vi "Robot Global Data.vi"() -> ()   [LabVIEW 2015]
doc: "This global VI can contain as many global variables as you need. Place a control on the panel, give it a good name. To read or write to it from a VI, drag the icon to the diagram of that VI. You can also drag from the project. Click on the node to change which global you access. You shouldn't have multiple locations writing to a global or it will cause a race-condition."
uses:
  <vilib>/Rock Robotics/WPI/Camera/WPI_CameraImageSize.ctl
  <vilib>/Rock Robotics/WPI/DriverStation/WPI_DriverStationRobotMode2.ctl
  Common Code/Auton Command Cluster.ctl
  Common Code/Drivetrain Status Cluster.ctl
  Common Code/Drivetrain Modes.ctl
  Common Code/Dist Drive Status.ctl
  Common Code/Dashboard Communication/Dashboard Display Data.ctl
  Common Code/Auton File Lists.ctl
  Common Code/Encoder Values Super Cluster.ctl
  Common Code/Encoder Values.ctl
  Common Code/IMU Data.ctl
  navX-MXP Library/COMMON/TypeDefs/Value TypeDefs/navX NAVX_CAL_STATUS.ctl
  navX-MXP Library/COMMON/TypeDefs/Value TypeDefs/navX NAVX_OP_STATUS.ctl
  Common Code/Power and Diagnostic Data.ctl
  Common Code/Utilities/PDP Data.ctl
  Common Code/Utilities/PCM Data.ctl
  Common Code/Shooter State Cluster.ctl
  Common Code/Shooter State.ctl
  Common Code/Shoot Modes Enum.ctl
  Common Code/Shot Type.ctl
  Common Code/Intake Status Cluster.ctl
  Common Code/Intake Mode.ctl
  Common Code/Intake States.ctl
  Common Code/Ultrasonic Data.ctl
  Common Code/Climb Status Cluster.ctl
  Common Code/Major Loop Times.ctl
  Common Code/Dashboard Communication/Dashboard Control Data.ctl
  Common Code/Shooter Presets.ctl
  Common Code/Shot Presets.ctl
  Common Code/Encoder Control.ctl
  Common Code/Drivetrain Settings.ctl
  Common Code/Goal Vision Packet.ctl
  Common Code/Dashboard Drivetrain Command.ctl
  Common Code/Drivetrain Vision.ctl
  Common Code/Ball Tracking Command Cluster.ctl
  Common Code/Ball Vision Packet.ctl
  Common Code/Tracking Mode.ctl
  Common Code/Intake Presets.ctl
  Common Code/Drivetrain Output Range.ctl
  Common Code/IntakeEcoderControl.ctl
  Common Code/Climb Presets.ctl
  Common Code/Shooter Command Cluster.ctl
  Common Code/Shooter Commands.ctl
  Common Code/Climb Command Cluster.ctl
  Common Code/Climb Mode.ctl
  Common Code/Climb Manual State.ctl
  Common Code/Drivetrain Commands.ctl
  Common Code/Manual Shoot.ctl
  Common Code/Intake Commands Cluster.ctl
  Common Code/Intake Commands.ctl
  Common Code/Manual Intake Commands.ctl
  Common Code/Keyboard Packet.ctl
  navX-MXP Library/navX-MXP IMU.lvlib
panel:
  in  "Right RPM":dbl
  in  "Left RPM":dbl
  out "Auton File Loop Timer":u32
  out "US Loop Timer":u32
  out "Intake Loop Timer":u32
  out "Shooter Loop Timer":u32
  out "DT Loop Timer":u32
  out "Climb Status Cluster":T1
  out "Ultrasonic Data":T2
  in  "Keyboard Cluster":T3
  out "Shooter State":T4 {"Trigger Output" scale=-1.0..1.0; "Angle Motor Output" scale=-1.0..1.0; "Right RPM" scale=0.0..5000.0; "Left RPM" scale=0.0..5000.0}
  in  "Intake Status Cluster":T8={"Roller Power"=0.0, "Angle Power"=0.0, "Intake Mode"=enum."Auto", "Intake States"=enum."Idle", "Rollers Active?"=FALSE, "Current Height"=0.0, "Target Height"=0.0, "Encoder Raw Position"=0.0, "Forward Tripped?"=FALSE, "Backward Tripped?"=FALSE, "Override IR?"=FALSE}
  out "Is IMU Reset?":bool
  in  "Reset IMU":bool
  in  "Boolean":bool
  in  "Intake Commands Cluster":T11={"Intake Commands"=enum."Load", "Intake Mode"=enum."Auto", "Override IR"=FALSE}
  in  "Manual Intake Commands":T13
  in  "Queue File Names":string[](array[string])
  in  "NavX Opened":bool
  in  "IMU Yaw Zero":dbl
  in  "IMU Roll Zero":dbl
  in  "IMU Pitch Zero":dbl
  in  "Manual Shoot":T14
  out "IMU Data":T15 {"NAVX_OP_STATUS" items=["INITIALIZING", "SELFTEST_IN_PROGRESS", "ERROR", "IMU_AUTOCAL_IN_PROGRESS", "NORMAL"]; "NAVX_CAL_STATUS" items=["IMU_CAL_STATE_MASK"=3, "IMU_CAL_INPROGRESS"=0, "IMU_CAL_ACCUMULATE"=1, "IMU_CAL_COMPLETE"=2, "MAG_CAL_COMPLETE"=4, "BARO_CAL_COMPLETE"=8]}
  in  "Right Pot 0":dbl
  in  "Left Pot 0":dbl
  out "Encoder Values":T18
  in  "Dashboard Drivetrain Command":T20
  out "General Scripts":string
  in  "Auton File Lists":T22
  in  "Current Auton Command Data":T23
  in  "Dashboard Packet":T24={"Shooter Presets"={"Batter Shot"={"Left Wheel RPM"=0.0, "Right Wheel RPM"=0.0, "Angle"=0.0}, "Deep Middle Shot"={"Left Wheel RPM"=0.0, "Right Wheel RPM"=0.0, "Angle"=0.0}, "Manual Shot"={"Left Wheel RPM"=0.0, "Right Wheel RPM"=0.0, "Angle"=0.0}, "Left Ticks Per Rotation"=0.0, "Right Ticks Per Rotation"=0.0, "Low Bar Shot"={"Left Wheel RPM"=0.0, "Right Wheel RPM"=0.0, "Angle"=0.0}, "Shooter RPM Tolerance"=0.0, "IIR Filter Power"=0.0, "Trigger Power"=0.0, "Fire from Load Delay"=0, "Angle Pot M"=0.0, "Angle Pot B"=0.0, "Shooter Length"=0.0, "String Pot Dist"=0.0, "Angle PID gains"={"proportional gain (Kc)"=1.0, "integral time (Ti, min)"=0.01, "derivative time (Td, min)"=0.0}, "Angle Motor Output"={"output high"=0.0, "output low"=0.0}, "Shooter Angle Tolerance"=0.0, "Vision Shoot x^2"=0.0, "Vision Shoot x"=0.0, "Dist from Axis Cam to Pivot"=0.0, "High Goal Center Height"=97.0, "Feed Forward Max Accel"=0.0, "Feed Forward Kv"=0.0, "Backwards Trigger"=0.0, "Shot Finish Delay (ms)"=0.0, "Angle Max Current"=0.0, "Angle Current Trip Time"=0.0, "Shooter Intake Angle"=0.0, "Vision Shoot c"=0.0, "Reset?"=FALSE, "Servo Release Delay"=0.0, "Servo Idle Angle"=0, "Servo Hold Angle"=0, "Angle Pot x^2"=0.0, "Angle Pot x"=0.0, "Angle Pot c"=0.0, "Ignore Angle?"=FALSE}, "Encoder Control"={"Right Tick Constant"=0.0, "Left Tick Constant"=0.0, "Reset?"=FALSE, "Y Dist"={"PID gains"={"proportional gain (Kc)"=0.0, "integral time (Ti, min)"=0.0, "derivative time (Td, min)"=0.0}}, "Y Stop Thresh"=0.0, "Y Stop Speed"=0.0}, "Steer PID output"={"output high"=0.0, "output low"=0.0}, " Steer PID gains"={"proportional gain (Kc)"=0.0, "integral time (Ti, min)"=0.0, "derivative time (Td, min)"=0.0}, "Drivetrain Settings"={"Gyro Tolerance"=0.0, "Throttle Ramp (ms)"=0.0, "Angular rate compensation"=FALSE, "Throttle to Rate Scale"=1.0, "Rate compensation gain"=0.01, "Kv"=0.0, "Ka"=0.0, "Feed Forward P"=0.0, "Feed Forward D"=0.0, "Goal Vision PID gains"={"proportional gain (Kc)"=1.0, "integral time (Ti, min)"=0.01, "derivative time (Td, min)"=0.0}, "Goal Detection Window"=0.0}, "Vision Packet"={"Distance"=0.0, "Center X"=0.0, "Center Y"=0.0, "Found Target?"=FALSE}, "Dashboard Drivetrain Command"={"Drivetrain Vision"={"Goal Window"=0.0, "Ball Window"=0.0}}, "Info/Command Cluster"={"Distance to Ball"=0.0, "Desired Angle"=0.0, "Command"=enum."Turn to Ball", "Pixels from Center"=0.0}, "Ball Vision Packet"={"Ball Detected?"=FALSE, "Distance to Ball"=0.0, "Desired Angle"=0.0, "Pixels from Center"=0.0, "Tracking mode"=enum."Turn to Ball"}, "Intake Presets"={"Intake Speed"=0.0, "Outake Speed"=0.0, "Low Height"=0.0, "Half Height"=0.0, "Full Height"=0.0, "Angle Speed"=0.0, "Fast Angle"=0.0, "Encoder Scale"=0.0, "Load Height"=0.0, "Output Range"={"output high"=0.0, "output low"=0.0}, "Rotation Power Max/Min"=0.0, "MaxCurrent"=0.0, "Intake Trip Time"=0.0, "Idle Height"=0.0, "Max Height"=0.0, "Reset Encoders?"=FALSE, "PID gains"={"proportional gain (Kc)"=0.0, "integral time (Ti, min)"=0.0, "derivative time (Td, min)"=0.0}}, "Intake Encoder Control"={"Arm Tick Constant"=0.0, "Reset?"=FALSE, "Y Dist"={"PID gains"={"proportional gain (Kc)"=0.0, "integral time (Ti, min)"=0.0, "derivative time (Td, min)"=0.0}}, "Y Stop Thresh"=0.0, "Y Stop Speed"=0.0}, "Climb Presets"={"Pull Power"=0.0, "Unpin Power"=0.0, "Time to Hold"=0.0}, "Ultrasonic Limit"=0.0, "Roll Limit"=0.0, "Pitch Limit"=0.0, "Goal Output Range"={"output high"=0.0, "output low"=0.0}} {"Intake Presets"."Max Height" format="%#_7g"; "Intake Presets"."Rotation Power Max/Min" format="%#_7g"; "Drivetrain Settings"."Goal Vision PID gains"."derivative time (Td, min)" format="%.3f"; "Drivetrain Settings"."Goal Vision PID gains"."integral time (Ti, min)" format="%.3f"; "Drivetrain Settings"."Goal Vision PID gains"."proportional gain (Kc)" format="%.3f"}
  out "Driver Station IP":dbl
  in  "Auton File Index":i32
  in  "Auton Field Index":i32
  out "Dashboard Status Data":T37={"Auton Command Cluster"={"Command ID"=0, "maxTime"=0.0, "Y Distance"=0.0, "Heading"=0.0, "Throttle"=0.0, "Async"=0.0, "Velocity"=0.0, "Acceleration"=0.0, "To"=0.0, "Condition"=0.0, "Shot Type"=0.0, "Left RPM"=0.0, "Override RPM"=0, "Override Angle"=0, "Right RPM"=0.0, "Angle"=0.0, "Intake Mode"=0, "Intake Cmd"=0, "Intake O"=0, "Eject O"=0, "Angle O"=0, "Arm O"=0, "Intake Speed"=0.0, "Eject Speed"=0.0, "Arm Angle"=0.0, "Arm Speed"=0.0, "Intake?"=0, "Eject?"=0}, "Auton File Lists"={"Current Queue"="", "General Scripts"="", "Defense Scripts"="", "Movement Scripts"=""}, "Drivetrain Status Cluster"={"Modes"=enum."Climb", "Y (Throttle)"=0.0, "X (Steer)"=0.0, "Gyro In Range?"=FALSE, "Distance Drive Finished?"=FALSE, "Stop Eject Lockout"=FALSE, "Dist Drive Status"={"Y In Range"=FALSE, "X In Range"=FALSE, "Gyro In Range"=FALSE, "Y Dist"=0.0, "X Dist"=0.0, "Gyro"=0.0}, "Y Target"=0.0, "Heading Target"=0.0, "Vision Target Aligned?"=FALSE, "Gear"=0.0, "1st Gear Time"=0.0, "2nd Gear Time"=0.0, "1st Gear Shifts"=0.0, "2nd Gear Shifts"=0.0}, "Encoder Values"={"Left Encoder"={"Distance"=0.0, "Speed"=0.0, "Ticks"=0.0}, "Right Encoder"={"Distance"=0.0, "Speed"=0.0, "Ticks"=0.0}}, "IMU Data"={"Pitch"=0.0, "Roll"=0.0, "Yaw"=0.0, "Data Valid?"=FALSE, "Temp"=0.0, "MOVING"=FALSE, "YAW_STABLE"=FALSE, "Accel X"=0.0, "Accel Y"=0.0, "Accel Z"=0.0, "Accel Magnitude"=0.0, "Pitch Rate"=0.0, "Roll Rate"=0.0, "Yaw Rate"=0.0, "NavX Opened?"=FALSE, "NAVX_CAL_STATUS"=0, "NAVX_OP_STATUS"=0}, "Power and Diagnostic Data"={"PDP Data"={"Battery Voltage"=0.0, "Temperature (degrees C)"=0.0, "Internal Battery R (Ohms)"=0.0, "Energy (J)"=0.0, "Power (W)"=0.0, "Total Current (A)"=0.0, "Battery Voltage Fault"=FALSE, "Temperature Fault"=FALSE, "Hardware Fault"=FALSE, "Currents"={"[0]"=0.0, "[1]"=0.0, "[2]"=0.0, "[3]"=0.0, "[4]"=0.0, "[5]"=0.0, "[6]"=0.0, "[7]"=0.0, "[8]"=0.0, "[9]"=0.0, "[10]"=0.0, "[11]"=0.0, "[12]"=0.0, "[13]"=0.0, "[14]"=0.0, "[15]"=0.0}, "Current Faults"={"[0]"=FALSE, "[1]"=FALSE, "[2]"=FALSE, "[3]"=FALSE, "[4]"=FALSE, "[5]"=FALSE, "[6]"=FALSE, "[7]"=FALSE, "[8]"=FALSE, "[9]"=FALSE, "[10]"=FALSE, "[11]"=FALSE, "[12]"=FALSE, "[13]"=FALSE, "[14]"=FALSE, "[15]"=FALSE}}, "PCM Data"={"Compressor Fault"=FALSE, "Solenoid Fault"=FALSE, "Compressor Enabled"=FALSE, "Hardware Fault"=FALSE, "Compressor Current"=0.0}, "roboRIO input voltage (V)"=0.0, "roboRIO input current (A)"=0.0, "3.3V Rail Short"=FALSE, "5 V Rail Short"=FALSE, "6 V Rail Short"=FALSE, "roboRIO Brownout"=FALSE, "Outputs Enabled?"=FALSE}, "Gyro"=0.0, "Shooter State Cluster"={"State"=enum."Idle", "Left RPM"=0.0, "Right RPM"=0.0, "Shooter Ready?"=FALSE, "Ball Loaded?"=FALSE, "Current Angle"=0.0, "Angle Motor Output"=0.0, "Trigger Output"=0.0, "Angle Ready?"=FALSE, "RPM Ready?"=FALSE, "Vision Ready?"=FALSE, "Ball Loaded?"=FALSE, "Mode"=enum."Manual", "Shot Type"=enum."Batter Shot", "Pot Height"=0.0, "Current Tripped Forward?"=FALSE, "Current Tripped Backward?"=FALSE, "Left Motor"=0.0, "Right Motor"=0.0, "Intake High?"=FALSE, "Raw Left Pos"=0.0, "Raw Right Pos"=0.0, "Raw Left V"=0.0, "Raw Right V"=0.0, "Right Servo"=0, "Left Servo"=0}, "Intake Status Cluster"={"Roller Power"=0.0, "Angle Power"=0.0, "Intake Mode"=enum."Auto", "Intake States"=enum."Idle", "Rollers Active?"=FALSE, "Current Height"=0.0, "Target Height"=0.0, "Encoder Raw Position"=0.0, "Forward Tripped?"=FALSE, "Backward Tripped?"=FALSE, "Override IR?"=FALSE}, "Ultrasonic Data"={"Left Ultrasonic"=0.0, "Right Ultrasonic"=0.0}, "Climb Status Cluster"={"Pull Power"=0.0, "Unpin Power"=0.0, "PTO Engaged?"=FALSE, "Pull Height"=0.0}, "Loop Times"={"DT Loop Timer"=0, "Shooter Loop Timer"=0, "Intake Loop Timer"=0, "US Loop Timer"=0, "Auton File Loop Timer"=0}} {"Shooter State Cluster"."Trigger Output" scale=-1.0..1.0; "Shooter State Cluster"."Angle Motor Output" scale=-1.0..1.0; "Shooter State Cluster"."Right RPM" scale=0.0..5000.0; "Shooter State Cluster"."Left RPM" scale=0.0..5000.0; "IMU Data"."NAVX_OP_STATUS" items=["INITIALIZING", "SELFTEST_IN_PROGRESS", "ERROR", "IMU_AUTOCAL_IN_PROGRESS", "NORMAL"]; "IMU Data"."NAVX_CAL_STATUS" items=["IMU_CAL_STATE_MASK"=3, "IMU_CAL_INPROGRESS"=0, "IMU_CAL_ACCUMULATE"=1, "IMU_CAL_COMPLETE"=2, "MAG_CAL_COMPLETE"=4, "BARO_CAL_COMPLETE"=8]; "Drivetrain Status Cluster"."2nd Gear Time" scale=0.0..135.0; "Drivetrain Status Cluster"."1st Gear Time" scale=0.0..135.0}
  in  "Auton File Build Loops":i32
  in  "Auton File Queue":path[](array[path])
  in  "Auton Command Array":T23[](array[typedef])
  in  "Shooter Commands":T45={"Command"=enum."Prime Shooter", "Mode"=enum."Manual", "Shot Type"=enum."Batter Shot", "Override Trigger IR"=FALSE, "Override Angle?"=FALSE}
  out "Drivetrain Status Cluster":T38={"Modes"=enum."Manual", "Y (Throttle)"=0.0, "X (Steer)"=0.0, "Gyro In Range?"=FALSE, "Distance Drive Finished?"=FALSE, "Stop Eject Lockout"=FALSE, "Dist Drive Status"={"Y In Range"=FALSE, "X In Range"=FALSE, "Gyro In Range"=FALSE, "Y Dist"=0.0, "X Dist"=0.0, "Gyro"=0.0}, "Y Target"=0.0, "Heading Target"=0.0, "Vision Target Aligned?"=FALSE, "Gear"=0.0, "1st Gear Time"=0.0, "2nd Gear Time"=0.0, "1st Gear Shifts"=0.0, "2nd Gear Shifts"=0.0} {"2nd Gear Time" scale=0.0..135.0; "1st Gear Time" scale=0.0..135.0}
  in  "Drivetrain Command Cluster":T47={"Y Power"=0.0, "Turn Power"=0.0, "1st Gear?"=FALSE, "Modes"=enum."Manual", "Heading Target"=0.0, "X Max Speed"=0.0, "Y Max Speed"=0.0, "X Min Speed"=0.0, "Y Min Speed"=0.0, "Y Target"=0.0, "Max Accel"=0.0, "Max Velocity"=0.0}
  in  "Robot Mode":T48
  in  "image size":T49=enum."320x240"
  in  "Enable Vision":bool
  in  "Climb Command Cluster":T50
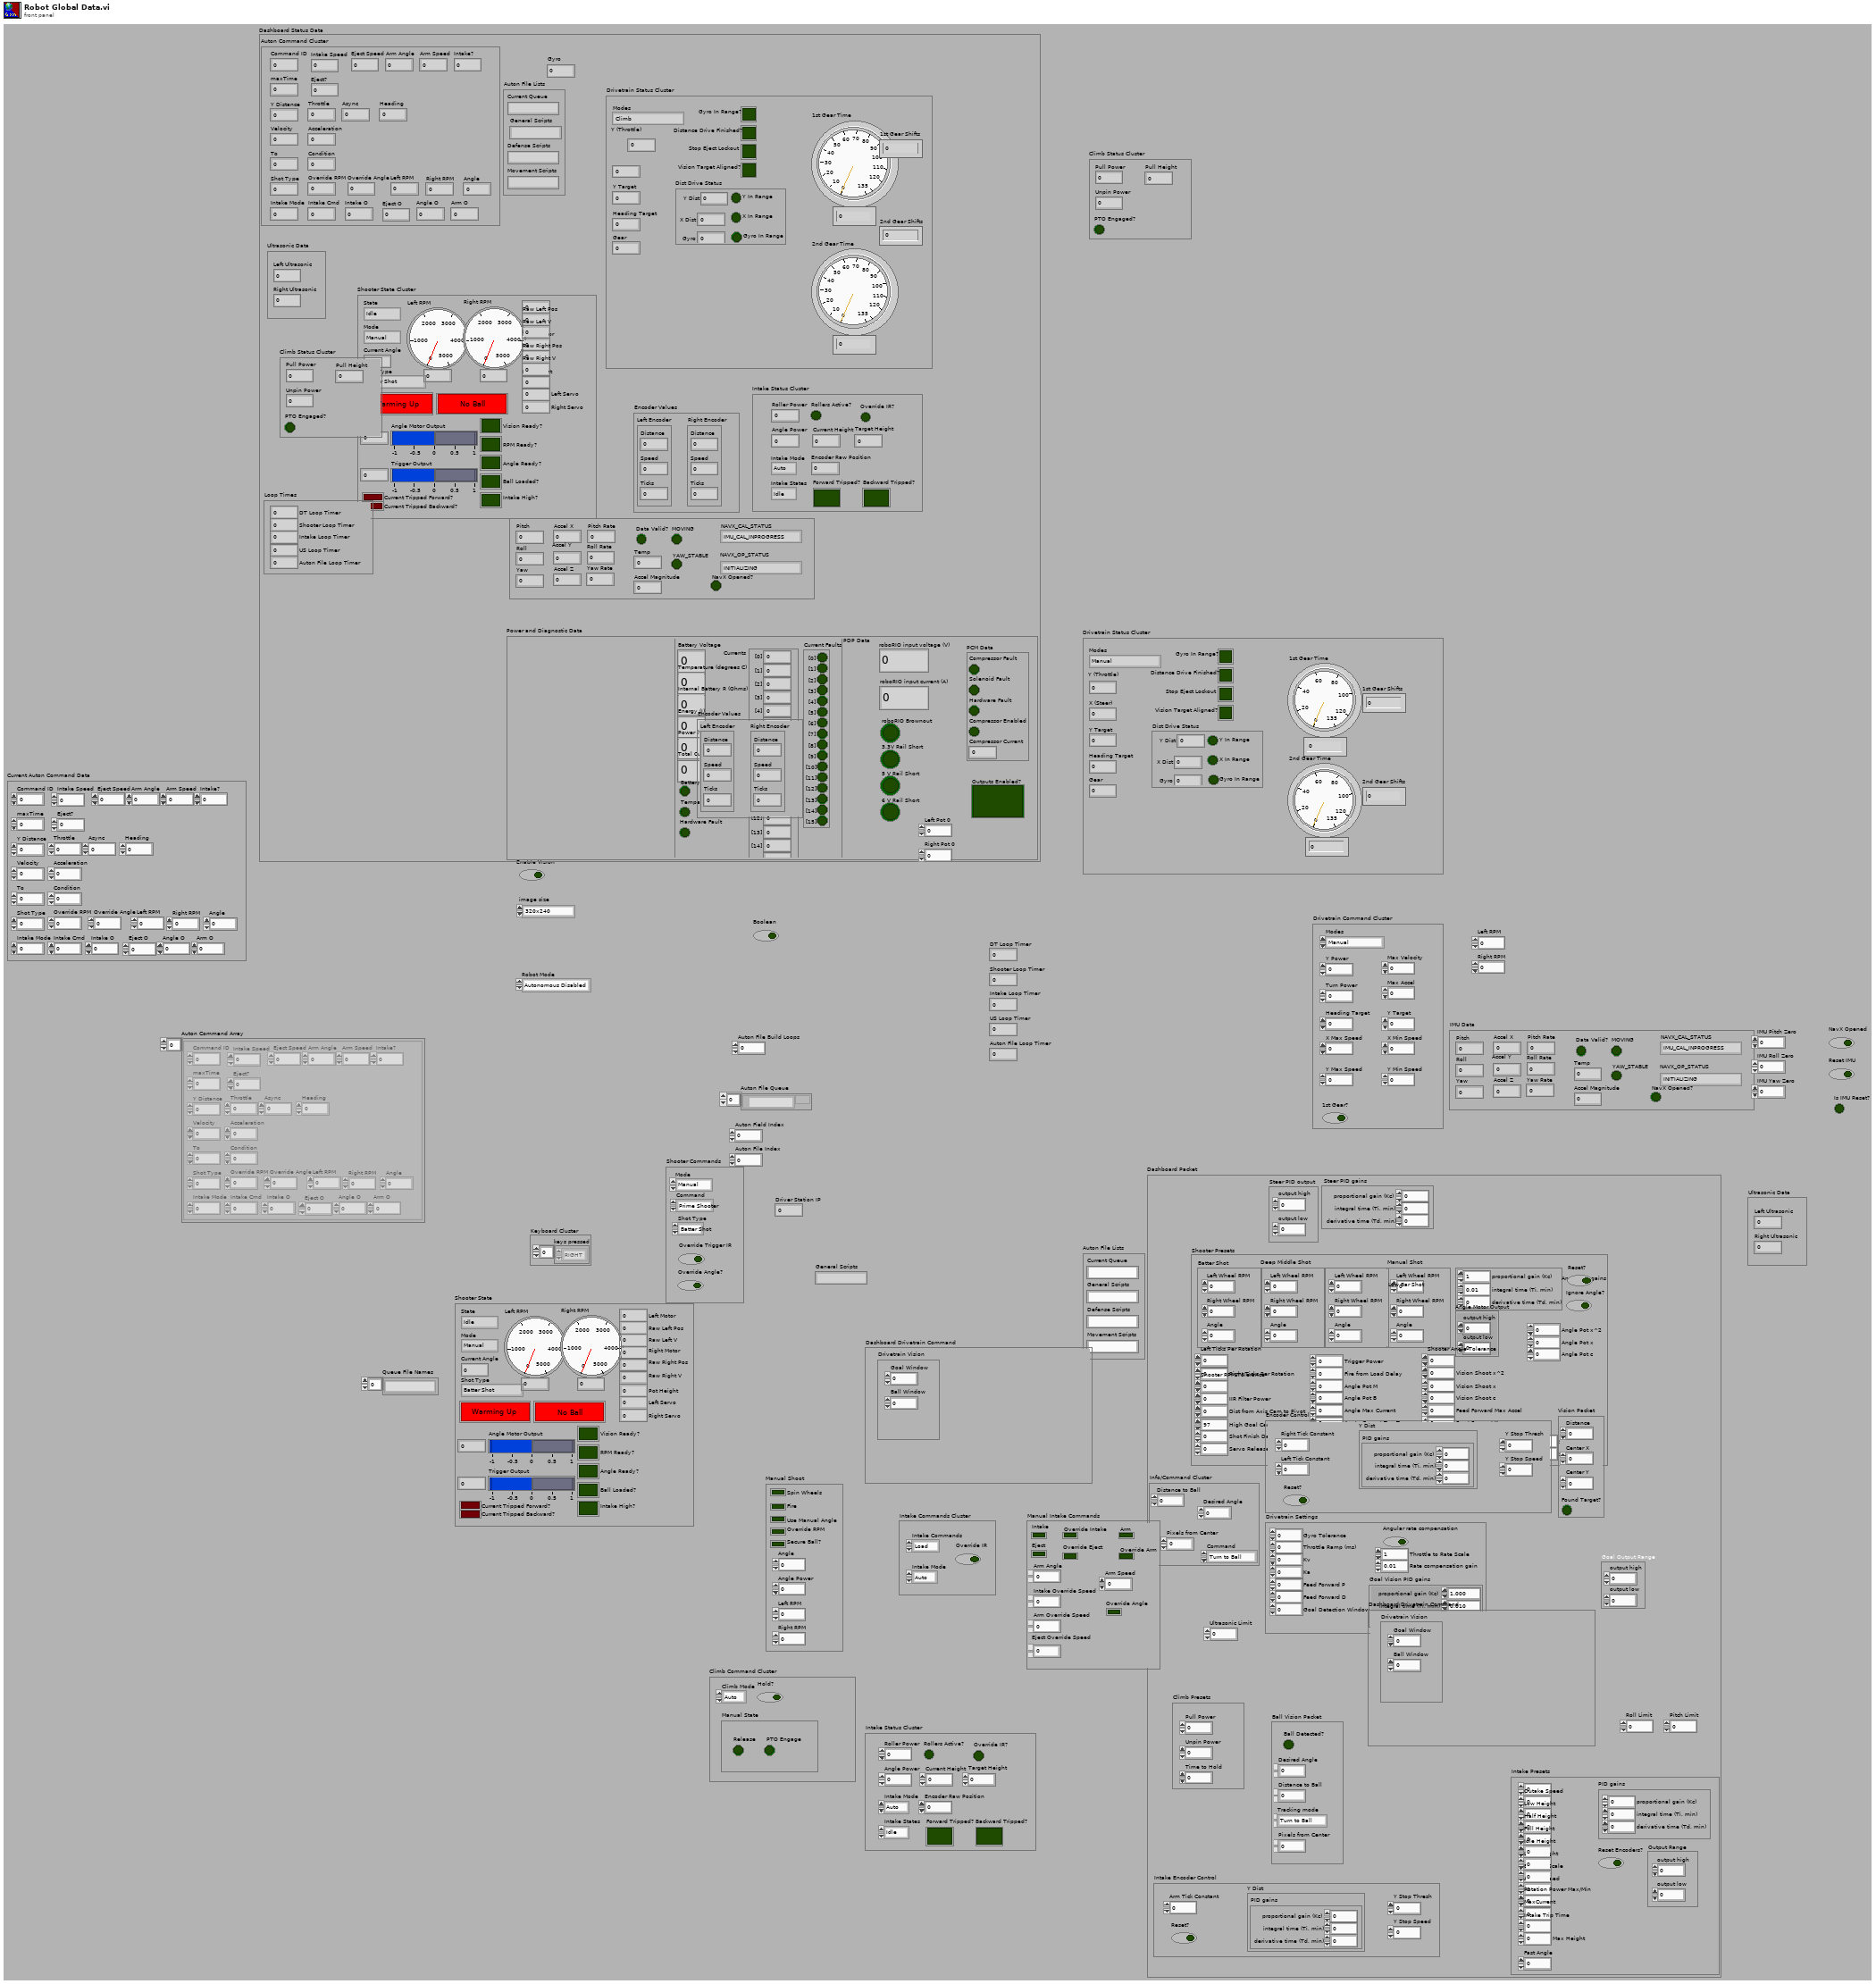
[diagram p1: front panel]
types:
  T1 = typedef "Climb Status Cluster.ctl" = cluster{"Pull Power":dbl, "Unpin Power":dbl, "PTO Engaged?":bool, "Pull Height":dbl}
  T2 = typedef "Ultrasonic Data.ctl" = cluster{"Left Ultrasonic":dbl, "Right Ultrasonic":dbl}
  T3 = typedef "Keyboard Packet.ctl" = cluster{"keys pressed":enum16{"0", "1", "2", "3", "4", "5", "6", "7", "8", "9", "A", "B", "C", "D", "E", "F", "G", "H", "I", "J", "K", "L", "M", "N", "O", "P", "Q", "R", "S", "T", "U", "V", "W", "X", "Y", "Z", "F1", "F2", "F3", "F4", "F5", "F6", "F7", "F8", "F9", "F10", "F11", "F12", "F13", "F14", "F15", "ADD", "BACK", "BACKSLASH", "CAPITAL", "COMMA", "DECIMAL", "DELETE", "DIVIDE", "DOWN", "END", "EQUALS", "ESCAPE", "GRAVE (`)", "HOME", "INSERT", "LBRACKET", "LCONTROL", "LEFT", "L ALT", "LSHIFT", "LWIN", "MINUS", "MULTIPLY", "NEXT", "NUMLOCK", "NUMPAD_0", "NUMPAD_1", "NUMPAD_2", "NUMPAD_3", "NUMPAD_4", "NUMPAD_5", "NUMPAD_6", "NUMPAD_7", "NUMPAD_8", "NUMPAD_9", "PAUSE", "PERIOD", "PRIOR (PG UP)", "RBRACKET", "RCONTROL", "RETURN", "RIGHT", "R ALT", "RSHIFT", "RWIN", "SCROLL", "SEMICOLON", "SLASH", "SPACE", "SUBTRACT", "TAB", "UP", "ENTER (num pad)", "' (quote)"}[]}
  T4 = typedef "Shooter State Cluster.ctl" = cluster{"State":T5, "Left RPM":dbl, "Right RPM":dbl, "Shooter Ready?":bool, "Ball Loaded?":bool, "Current Angle":dbl, "Angle Motor Output":dbl, "Trigger Output":dbl, "Angle Ready?":bool, "RPM Ready?":bool, "Vision Ready?":bool, "Ball Loaded?":bool, "Mode":T6, "Shot Type":T7, "Pot Height":dbl, "Current Tripped Forward?":bool, "Current Tripped Backward?":bool, "Left Motor":dbl, "Right Motor":dbl, "Intake High?":bool, "Raw Left Pos":dbl, "Raw Right Pos":dbl, "Raw Left V":dbl, "Raw Right V":dbl, "Right Servo":i32, "Left Servo":i32}
  T5 = typedef "Shooter State.ctl" = enum16{"Idle", "Warmup", "Shooter Ready", "Shoot"}
  T6 = typedef "Shoot Modes Enum.ctl" = enum16{"Manual", "Safe", "Auto"}
  T7 = typedef "Shot Type.ctl" = enum16{"Batter Shot", "Corner Shot", "Curve Shot", "Vision Shot", "Deep Middle Shot"}
  T8 = typedef "Intake Status Cluster.ctl" = cluster{"Roller Power":dbl, "Angle Power":dbl, "Intake Mode":T9, "Intake States":T10, "Rollers Active?":bool, "Current Height":dbl, "Target Height":dbl, "Encoder Raw Position":dbl, "Forward Tripped?":bool, "Backward Tripped?":bool, "Override IR?":bool}
  T9 = typedef "Intake Mode.ctl" = enum16{"Safe", "Auto", "Manual"}
  T10 = typedef "Intake States.ctl" = enum16{"Idle", "Set roller speed", "Move to angle"}
  T11 = typedef "Intake Commands Cluster.ctl" = cluster{"Intake Commands":T12, "Intake Mode":T9, "Override IR":bool}
  T12 = typedef "Intake Commands.ctl" = enum16{"Unload", "Load", "Pull up", "Drop low", "Idle", "Lift Half"}
  T13 = typedef "Manual Intake Commands.ctl" = cluster{"Intake":bool, "Eject":bool, "Arm Angle":dbl, "Intake Override Speed":dbl, "Arm Override Speed":dbl, "Arm Speed":dbl, "Override Intake":bool, "Override Eject":bool, "Eject Override Speed":dbl, "Arm":bool, "Override Arm":bool, "Override Angle":bool}
  T14 = typedef "Manual Shoot.ctl" = cluster{"Spin Wheels":bool, "Fire":bool, "Angle":dbl, "Angle Power":dbl, "Use Manual Angle":bool, "Override RPM":bool, "Left RPM":dbl, "Right RPM":dbl, "Secure Ball?":bool}
  T15 = typedef "IMU Data.ctl" = cluster{"Pitch":sgl, "Roll":sgl, "Yaw":sgl, "Data Valid?":bool, "Temp":sgl, "MOVING":bool, "YAW_STABLE":bool, "Accel X":sgl, "Accel Y":sgl, "Accel Z":sgl, "Accel Magnitude":sgl, "Pitch Rate":sgl, "Roll Rate":sgl, "Yaw Rate":sgl, "NavX Opened?":bool, "NAVX_CAL_STATUS":T16, "NAVX_OP_STATUS":T17}
  T16 = typedef "navX-MXP IMU.lvlib/navX NAVX_CAL_STATUS.ctl" = u8
  T17 = typedef "navX-MXP IMU.lvlib/navX NAVX_OP_STATUS.ctl" = u8
  T18 = typedef "Encoder Values Super Cluster.ctl" = cluster{"Left Encoder":T19, "Right Encoder":T19}
  T19 = typedef "Encoder Values.ctl" = cluster{"Distance":dbl, "Speed":dbl, "Ticks":dbl}
  T20 = typedef "Dashboard Drivetrain Command.ctl" = cluster{"Drivetrain Vision":T21}
  T21 = typedef "Drivetrain Vision.ctl" = cluster{"Goal Window":dbl, "Ball Window":dbl}
  T22 = typedef "Auton File Lists.ctl" = cluster{"Current Queue":string, "General Scripts":string, "Defense Scripts":string, "Movement Scripts":string}
  T23 = typedef "Auton Command Cluster.ctl" = cluster{"Command ID":i32, "maxTime":dbl, "Y Distance":dbl, "Heading":dbl, "Throttle":dbl, "Async":dbl, "Velocity":dbl, "Acceleration":dbl, "To":dbl, "Condition":dbl, "Shot Type":dbl, "Left RPM":dbl, "Override RPM":i32, "Override Angle":i32, "Right RPM":dbl, "Angle":dbl, "Intake Mode":i32, "Intake Cmd":i32, "Intake O":i32, "Eject O":i32, "Angle O":i32, "Arm O":i32, "Intake Speed":dbl, "Eject Speed":dbl, "Arm Angle":dbl, "Arm Speed":dbl, "Intake?":i32, "Eject?":i32}
  T24 = typedef "Dashboard Control Data.ctl" = cluster{"Shooter Presets":T25, "Encoder Control":T27, "Steer PID output":cluster{"output high":dbl, "output low":dbl}, " Steer PID gains":cluster{"proportional gain (Kc)":dbl, "integral time (Ti, min)":dbl, "derivative time (Td, min)":dbl}, "Drivetrain Settings":T28, "Vision Packet":T29, "Dashboard Drivetrain Command":T20, "Info/Command Cluster":T30, "Ball Vision Packet":T31, "Intake Presets":T33, "Intake Encoder Control":T35, "Climb Presets":T36, "Ultrasonic Limit":dbl, "Roll Limit":dbl, "Pitch Limit":dbl, "Goal Output Range":cluster{"output high":dbl, "output low":dbl}}
  T25 = typedef "Shooter Presets.ctl" = cluster{"Batter Shot":T26, "Deep Middle Shot":T26, "Manual Shot":T26, "Left Ticks Per Rotation":dbl, "Right Ticks Per Rotation":dbl, "Low Bar Shot":T26, "Shooter RPM Tolerance":dbl, "IIR Filter Power":dbl, "Trigger Power":dbl, "Fire from Load Delay":i32, "Angle Pot M":dbl, "Angle Pot B":dbl, "Shooter Length":dbl, "String Pot Dist":dbl, "Angle PID gains":cluster{"proportional gain (Kc)":dbl, "integral time (Ti, min)":dbl, "derivative time (Td, min)":dbl}, "Angle Motor Output":cluster{"output high":dbl, "output low":dbl}, "Shooter Angle Tolerance":dbl, "Vision Shoot x^2":dbl, "Vision Shoot x":dbl, "Dist from Axis Cam to Pivot":dbl, "High Goal Center Height":dbl, "Feed Forward Max Accel":dbl, "Feed Forward Kv":dbl, "Backwards Trigger":dbl, "Shot Finish Delay (ms)":dbl, "Angle Max Current":dbl, "Angle Current Trip Time":dbl, "Shooter Intake Angle":dbl, "Vision Shoot c":dbl, "Reset?":bool, "Servo Release Delay":dbl, "Servo Idle Angle":i32, "Servo Hold Angle":i32, "Angle Pot x^2":dbl, "Angle Pot x":dbl, "Angle Pot c":dbl, "Ignore Angle?":bool}
  T26 = typedef "Shot Presets.ctl" = cluster{"Left Wheel RPM":dbl, "Right Wheel RPM":dbl, "Angle":dbl}
  T27 = typedef "Encoder Control.ctl" = cluster{"Right Tick Constant":dbl, "Left Tick Constant":dbl, "Reset?":bool, "Y Dist":cluster{"PID gains":cluster{"proportional gain (Kc)":dbl, "integral time (Ti, min)":dbl, "derivative time (Td, min)":dbl}}, "Y Stop Thresh":dbl, "Y Stop Speed":dbl}
  T28 = typedef "Drivetrain Settings.ctl" = cluster{"Gyro Tolerance":dbl, "Throttle Ramp (ms)":dbl, "Angular rate compensation":bool, "Throttle to Rate Scale":dbl, "Rate compensation gain":dbl, "Kv":dbl, "Ka":dbl, "Feed Forward P":dbl, "Feed Forward D":dbl, "Goal Vision PID gains":cluster{"proportional gain (Kc)":dbl, "integral time (Ti, min)":dbl, "derivative time (Td, min)":dbl}, "Goal Detection Window":dbl}
  T29 = typedef "Goal Vision Packet.ctl" = cluster{"Distance":dbl, "Center X":dbl, "Center Y":dbl, "Found Target?":bool}
  T30 = typedef "Ball Tracking Command Cluster.ctl" = cluster{"Distance to Ball":dbl, "Desired Angle":dbl, "Command":enum16{"Turn to Ball", "Turn to Angle", "Get Distance"}, "Pixels from Center":dbl}
  T31 = typedef "Ball Vision Packet.ctl" = cluster{"Ball Detected?":bool, "Distance to Ball":dbl, "Desired Angle":dbl, "Pixels from Center":dbl, "Tracking mode":T32}
  T32 = typedef "Tracking Mode.ctl" = enum16{"Turn to Ball", "Turn to Angle"}
  T33 = typedef "Intake Presets.ctl" = cluster{"Intake Speed":dbl, "Outake Speed":dbl, "Low Height":dbl, "Half Height":dbl, "Full Height":dbl, "Angle Speed":dbl, "Fast Angle":dbl, "Encoder Scale":dbl, "Load Height":dbl, "Output Range":T34, "Rotation Power Max/Min":dbl, "MaxCurrent":dbl, "Intake Trip Time":dbl, "Idle Height":dbl, "Max Height":dbl, "Reset Encoders?":bool, "PID gains":cluster{"proportional gain (Kc)":dbl, "integral time (Ti, min)":dbl, "derivative time (Td, min)":dbl}}
  T34 = typedef "Drivetrain Output Range.ctl" = cluster{"output high":dbl, "output low":dbl}
  T35 = typedef "IntakeEcoderControl.ctl" = cluster{"Arm Tick Constant":dbl, "Reset?":bool, "Y Dist":cluster{"PID gains":cluster{"proportional gain (Kc)":dbl, "integral time (Ti, min)":dbl, "derivative time (Td, min)":dbl}}, "Y Stop Thresh":dbl, "Y Stop Speed":dbl}
  T36 = typedef "Climb Presets.ctl" = cluster{"Pull Power":dbl, "Unpin Power":dbl, "Time to Hold":dbl}
  T37 = typedef "Dashboard Display Data.ctl" = cluster{"Auton Command Cluster":T23, "Auton File Lists":T22, "Drivetrain Status Cluster":T38, "Encoder Values":T18, "IMU Data":T15, "Power and Diagnostic Data":T41, "Gyro":dbl, "Shooter State Cluster":T4, "Intake Status Cluster":T8, "Ultrasonic Data":T2, "Climb Status Cluster":T1, "Loop Times":T44}
  T38 = typedef "Drivetrain Status Cluster.ctl" = cluster{"Modes":T39, "Y (Throttle)":dbl, "X (Steer)":dbl, "Gyro In Range?":bool, "Distance Drive Finished?":bool, "Stop Eject Lockout":bool, "Dist Drive Status":T40, "Y Target":dbl, "Heading Target":dbl, "Vision Target Aligned?":bool, "Gear":dbl, "1st Gear Time":dbl, "2nd Gear Time":dbl, "1st Gear Shifts":dbl, "2nd Gear Shifts":dbl}
  T39 = typedef "Drivetrain Modes.ctl" = enum16{"Climb", "Manual", "Ball Vision Targeting", "Goal Vision Targeting", "PID Distance Drive", "Hybrid"}
  T40 = typedef "Dist Drive Status.ctl" = cluster{"Y In Range":bool, "X In Range":bool, "Gyro In Range":bool, "Y Dist":dbl, "X Dist":dbl, "Gyro":dbl}
  T41 = typedef "Power and Diagnostic Data.ctl" = cluster{"PDP Data":T42, "PCM Data":T43, "roboRIO input voltage (V)":dbl, "roboRIO input current (A)":dbl, "3.3V Rail Short":bool, "5 V Rail Short":bool, "6 V Rail Short":bool, "roboRIO Brownout":bool, "Outputs Enabled?":bool}
  T42 = typedef "PDP Data.ctl" = cluster{"Battery Voltage":sgl, "Temperature (degrees C)":sgl, "Internal Battery R (Ohms)":sgl, "Energy (J)":sgl, "Power (W)":sgl, "Total Current (A)":sgl, "Battery Voltage Fault":bool, "Temperature Fault":bool, "Hardware Fault":bool, "Currents":cluster{"[0]":sgl, "[1]":sgl, "[2]":sgl, "[3]":sgl, "[4]":sgl, "[5]":sgl, "[6]":sgl, "[7]":sgl, "[8]":sgl, "[9]":sgl, "[10]":sgl, "[11]":sgl, "[12]":sgl, "[13]":sgl, "[14]":sgl, "[15]":sgl}, "Current Faults":cluster{"[0]":bool, "[1]":bool, "[2]":bool, "[3]":bool, "[4]":bool, "[5]":bool, "[6]":bool, "[7]":bool, "[8]":bool, "[9]":bool, "[10]":bool, "[11]":bool, "[12]":bool, "[13]":bool, "[14]":bool, "[15]":bool}}
  T43 = typedef "PCM Data.ctl" = cluster{"Compressor Fault":bool, "Solenoid Fault":bool, "Compressor Enabled":bool, "Hardware Fault":bool, "Compressor Current":dbl}
  T44 = typedef "Major Loop Times.ctl" = cluster{"DT Loop Timer":u32, "Shooter Loop Timer":u32, "Intake Loop Timer":u32, "US Loop Timer":u32, "Auton File Loop Timer":u32}
  T45 = typedef "Shooter Command Cluster.ctl" = cluster{"Command":T46, "Mode":T6, "Shot Type":T7, "Override Trigger IR":bool, "Override Angle?":bool}
  T46 = typedef "Shooter Commands.ctl" = enum16{"Idle", "Prime Shooter", "Shoot"}
  T47 = typedef "Drivetrain Commands.ctl" = cluster{"Y Power":dbl, "Turn Power":dbl, "1st Gear?":bool, "Modes":T39, "Heading Target":dbl, "X Max Speed":dbl, "Y Max Speed":dbl, "X Min Speed":dbl, "Y Min Speed":dbl, "Y Target":dbl, "Max Accel":dbl, "Max Velocity":dbl}
  T48 = typedef "WPI_DriverStationRobotMode2.ctl" = enum16{"Autonomous Disabled", "Autonomous Enabled", "Teleop Disabled", "Teleop Enabled", "Disconnected", "Finish", "Test Disabled", "Test Enabled", "Emergency Stopped"}
  T49 = typedef "WPI_CameraImageSize.ctl" = enum16{"640x480", "320x240", "160x120", "Custom"}
  T50 = typedef "Climb Command Cluster.ctl" = cluster{"Climb Mode":T51, "Hold?":bool, "Manual State":T52}
  T51 = typedef "Climb Mode.ctl" = enum16{"Auto", "Manual"}
  T52 = typedef "Climb Manual State.ctl" = cluster{"Release":bool, " PTO Engage":bool}
diagram:
